vi "SiPM_Data_Analysis.vi"() -> ()   [LabVIEW 2019]
uses:
  <vilib>/Utility/error.llb/DialogType.ctl
  SiPM_Tests_Global_Var.vi
  Data_Analysis_subvis/ESA_Data_Analysis_Global_VIs.vi
  <vilib>/Analysis/NI_AALPro.lvlib
panel:
  out "property names":string[](array[string])
  out "property values":variant[](array[variant])
  out "data":waveform(dbl)[](array[waveform])
  out "Indicator":bool
  in  "Close Session":bool
  in  "Channel Selection":T1(ring)=enum."Channel 6"
  in  "Waveform Nb":u16
  in  "NbSamples":i64=1000000 caption="Nb of Samples to Analyze" format="%.0p"
  in  "Refresh":bool
  in  "Load file to display":bool
  in  "Detailed":bool
  in  "Listbox":i32[](listbox) caption="PIFN_ReadoutBoard.tdms"
  in  "CH6 Trigger Logic":T2(ring)=enum."Don't Care"
  in  "CH6 Trigger Thr":u16 caption="CH6 Trigger Thr (V)" step=1
  in  "CH5 Trigger Logic":T2(ring)=enum."Don't Care"
  in  "CH5 Trigger":u16 caption="CH5 Trigger Thr (V)" step=1
  in  "Tab Control":enum32{"Waveform", "Calibration"}(tab)
  out "Spectrum":u16[][](graph)
  in  "X-Scale":bool
  in  "Calibrate":bool
  out "Offset":dbl step=0.001 format="%#_6p"
  out "Gain":dbl step=0.001 format="%#_6p"
  in  "Y2 (keV)":dbl
  in  "Y1 (keV)":dbl
  in  "AutoScale 4":bool
  out "Waveform Graph":dbl[][](graph)
  in  "Lower Cut-Off":dbl=0.01
  in  "Y-Scale 2":bool caption="Y-Scale"
  in  "CH1 Trigger Logic":T2(ring)=enum."Don't Care"
  in  "CH1 Trigger Thr":u16 caption="CH1 Trigger Thr (V)" step=1
  in  "Y-Scale":bool
  out "Nb of Selected Events":dbl step=0.001 format="%#_6p"
  out "Total Nb of Recorded Events":dbl step=0.001 format="%#_6p"
  in  "CH4 Trigger Logic":T2(ring)=enum."Don't Care"
  in  "CH4 Trigger Thr":u16 caption="CH4 Trigger Thr (V)" step=1
  in  "CH3 Trigger Logic":T2(ring)=enum."Don't Care"
  in  "CH3 Trigger":u16 caption="CH3 Trigger Thr (V)" step=1
  in  "CH2 Trigger Logic":T2(ring)=enum."Don't Care"
  in  "CH2 Trigger Thr":u16 caption="CH2 Trigger Thr (V)" step=1
  in  "AutoScale 3":bool
  in  "Update Energy":bool
  out "Energy_Spectr":u16[][](graph)
  in  "Filter \nON?":bool
  in  "Threshold 2":dbl caption="Max_Value (V)" step=0.001 format="%#_6p"
  in  "Threshold":dbl caption="Energy Threshold (V)" step=0.001 format="%#_6p"
  out "Table":string[][](table)
  out "Nb of Channels in Group":i32
  out "group names":string[](array[string])
  out "tdms file out":refnum<k34>
  in  "File contents":string[](tree)
  # "NCSR  DEMOKRITOS\nInstitute of Nuclear and Particle Physics\nDetectors Instrumentation Laboratory"
  # "SiPM Data Analysis"
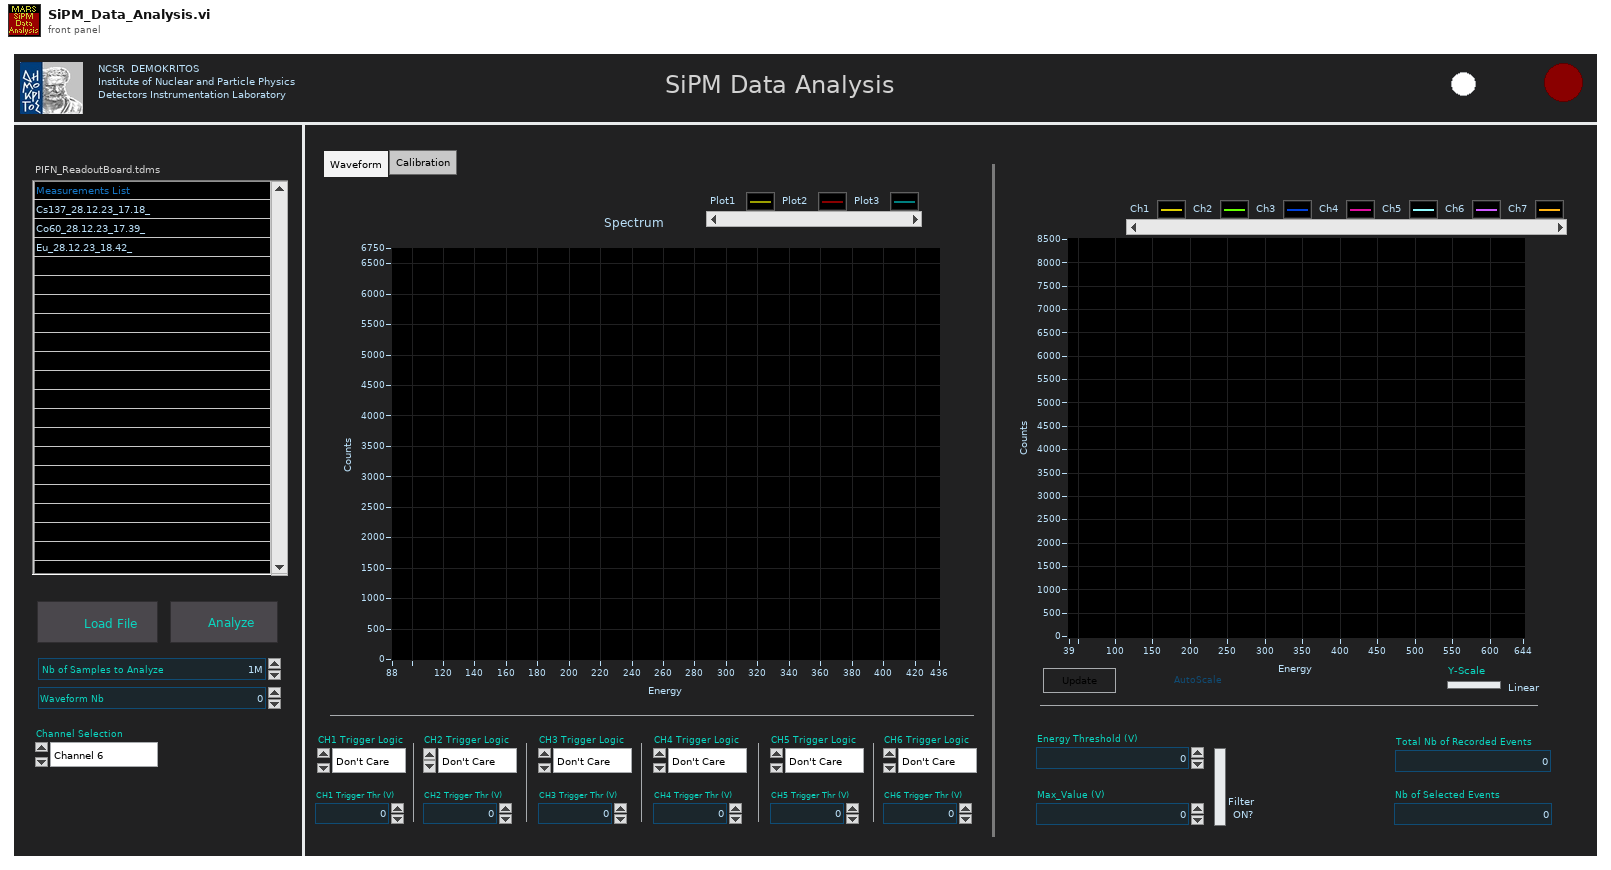
[diagram p1: front panel]
types:
  T1 = enum16{"Channel 1", "Channel 2", "Channel 3", "Channel 4", "Channle 5", "Channel 6", "Added Spectrum"}
  T2 = enum16{"Coincidence", "Anti-Coincidence", "Don't Care"}
  T3 = typedef "DialogType.ctl" = u16
  T4 = enum16{"open", "open or create", "create or replace", "create", "open (read-only)"}
  T5 = cluster{"X Values":dbl[], "Histogram: h(x)":i32[]}
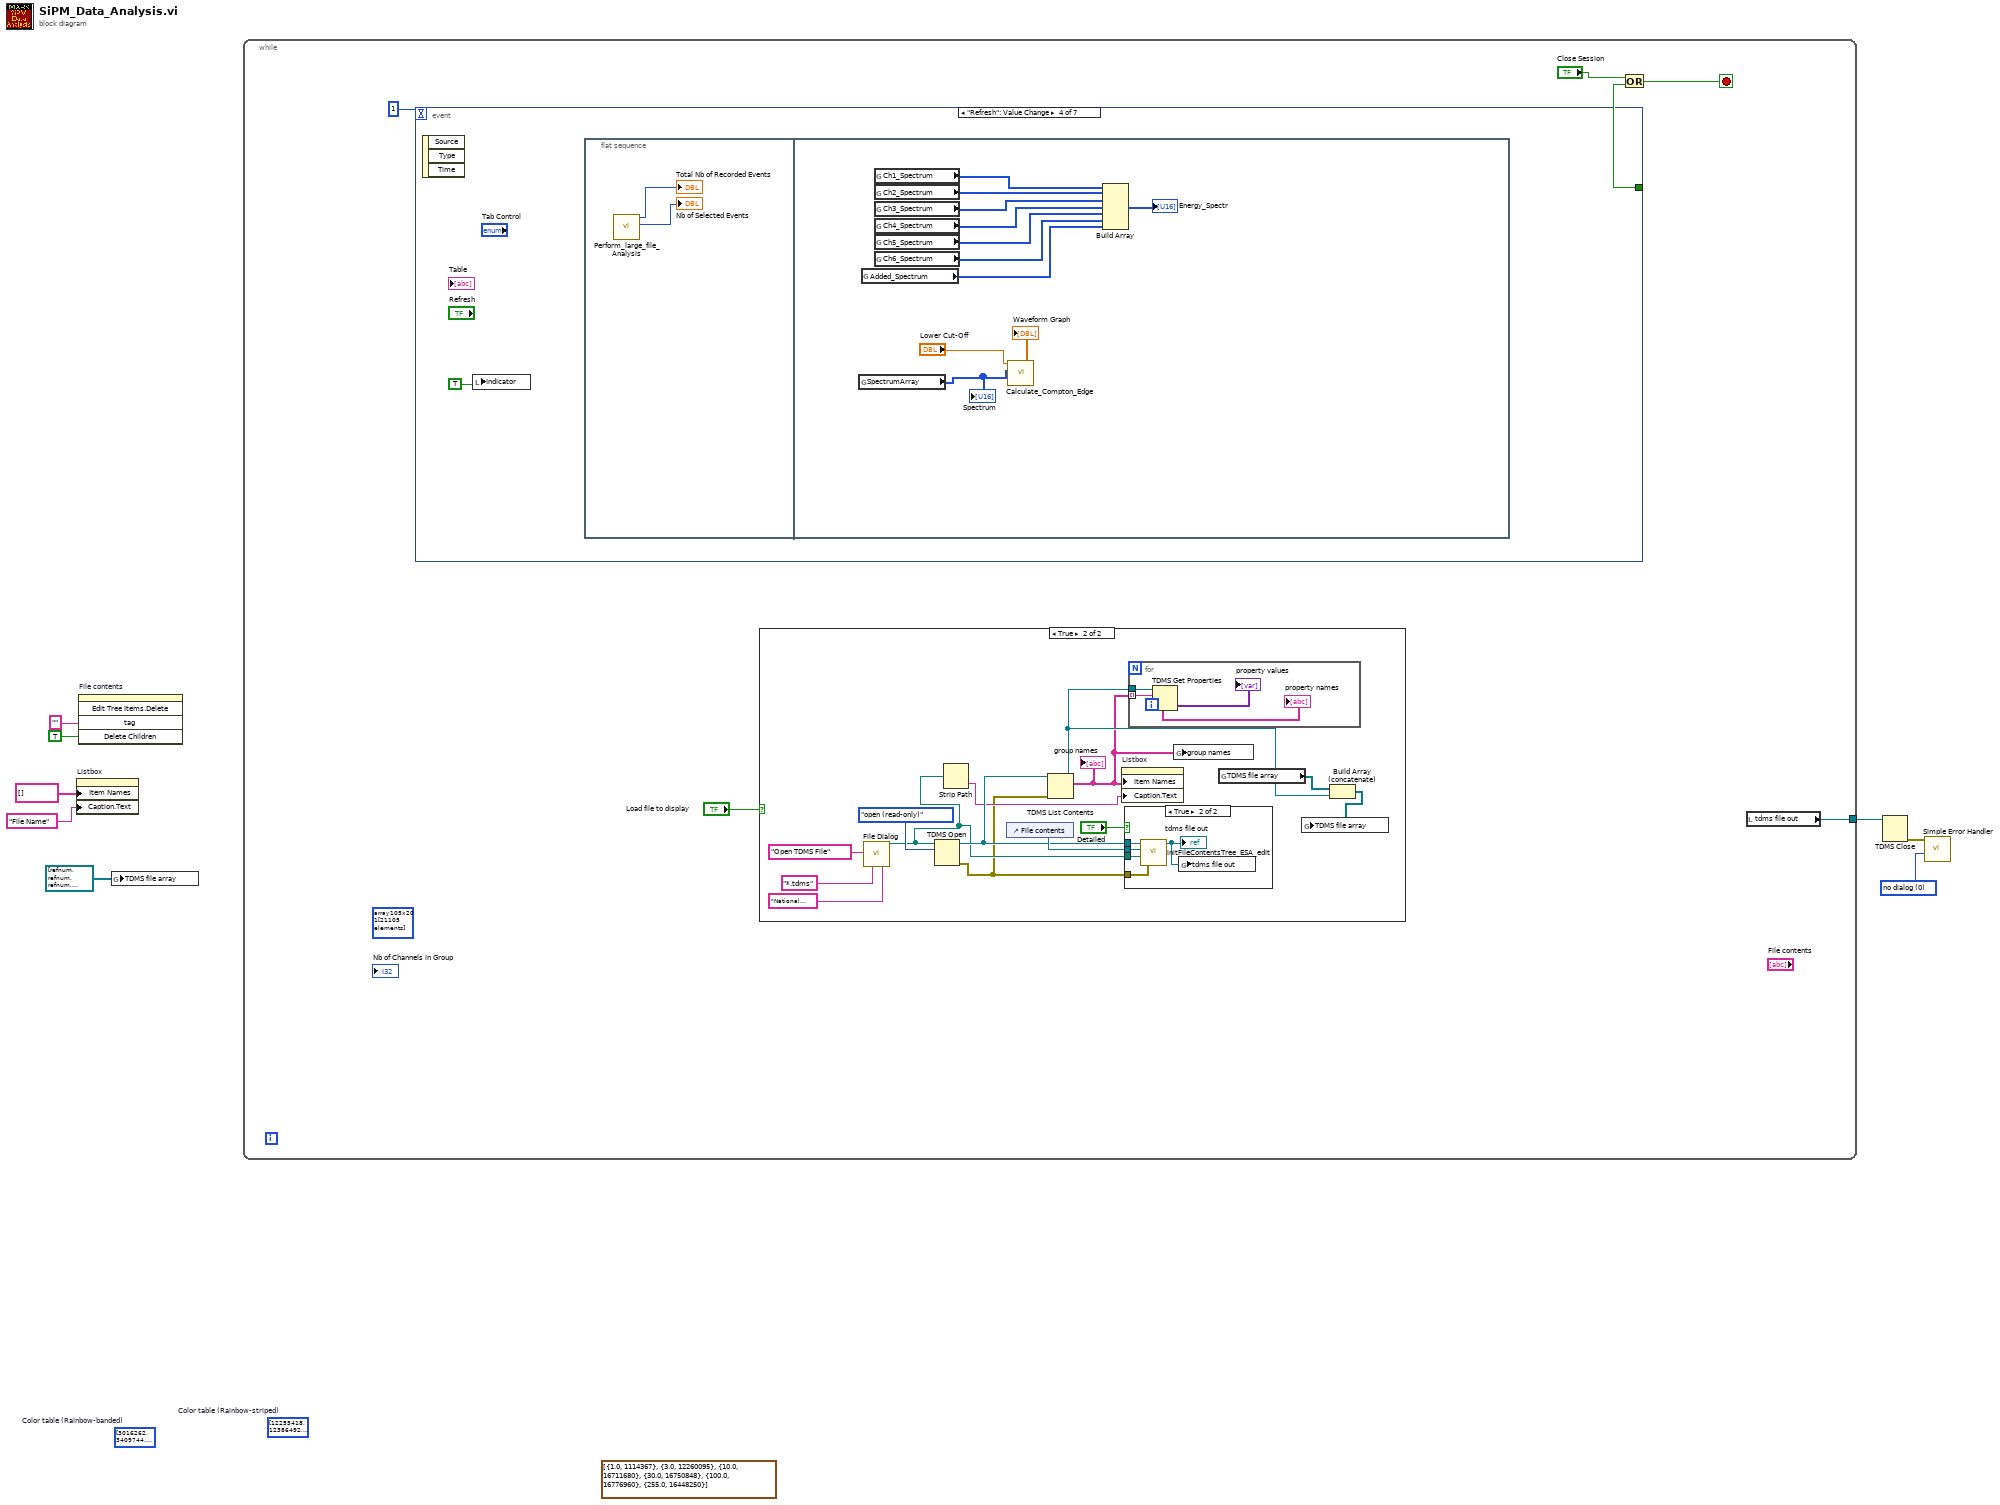
[diagram p0: block diagram]
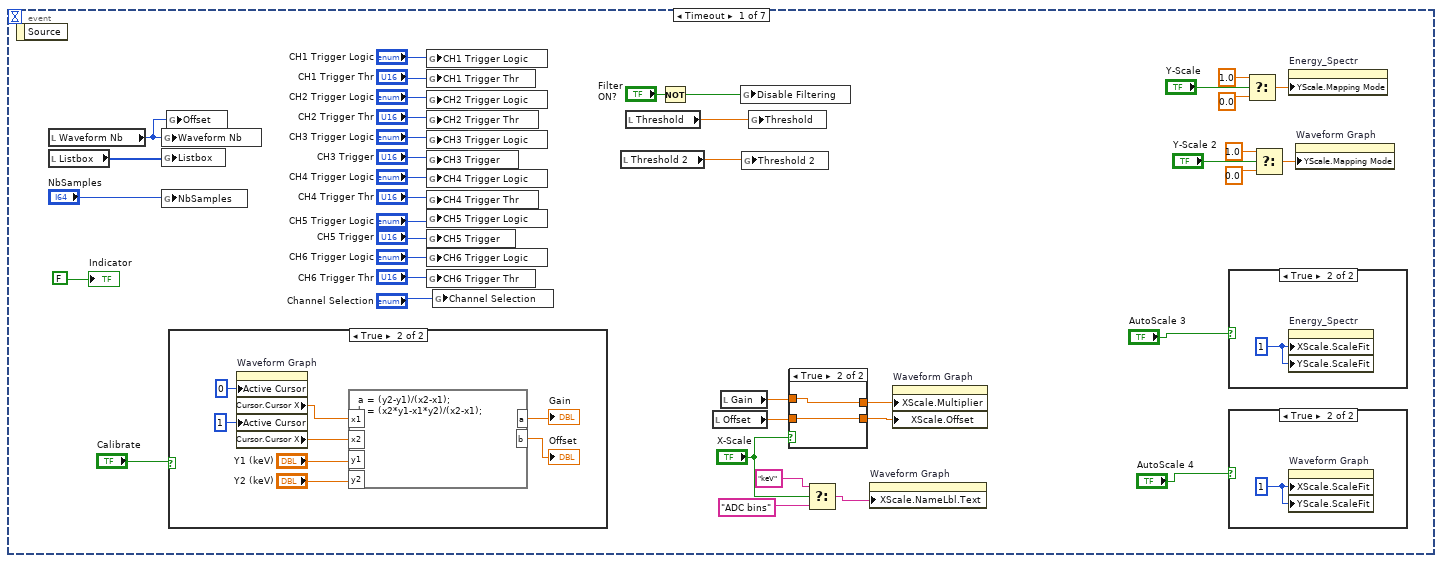
[diagram p2: hidden frame]
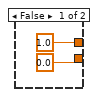
[diagram p3: hidden frame]
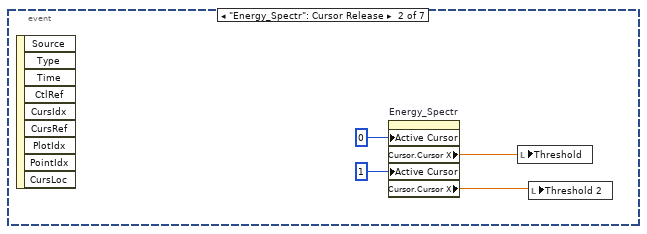
[diagram p7: hidden frame]
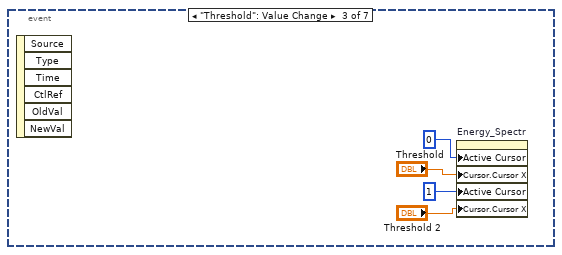
[diagram p8: hidden frame]
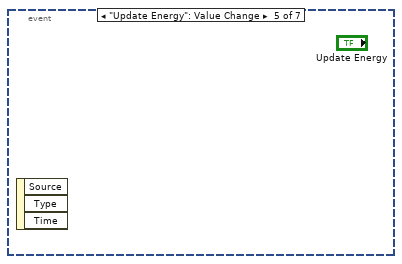
[diagram p9: hidden frame]
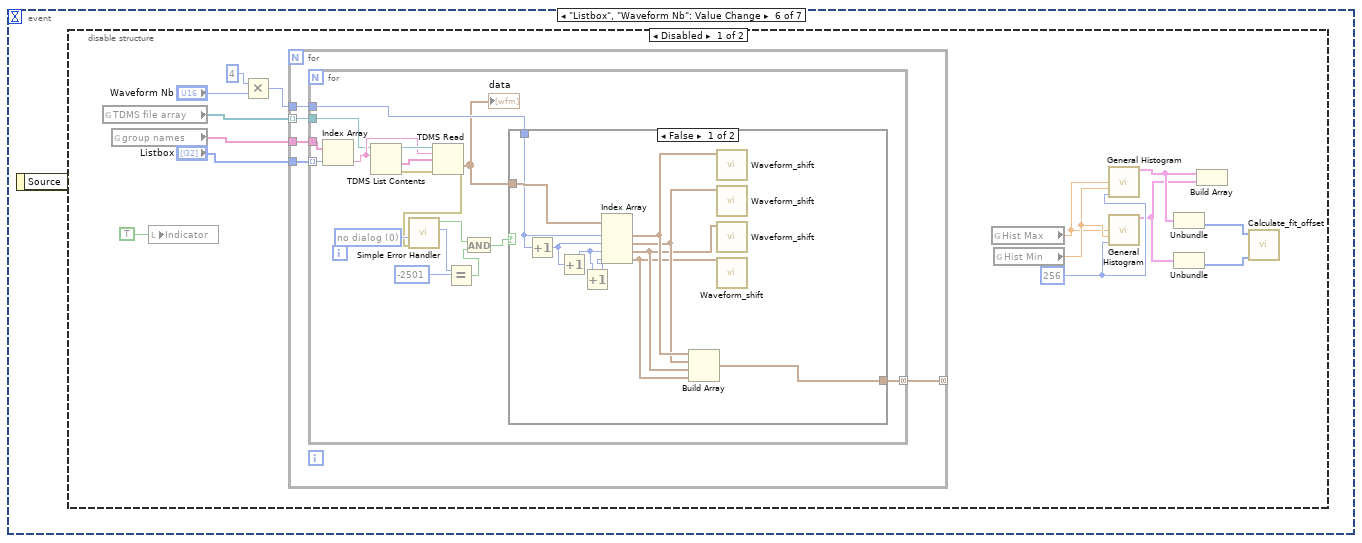
[diagram p10: hidden frame]
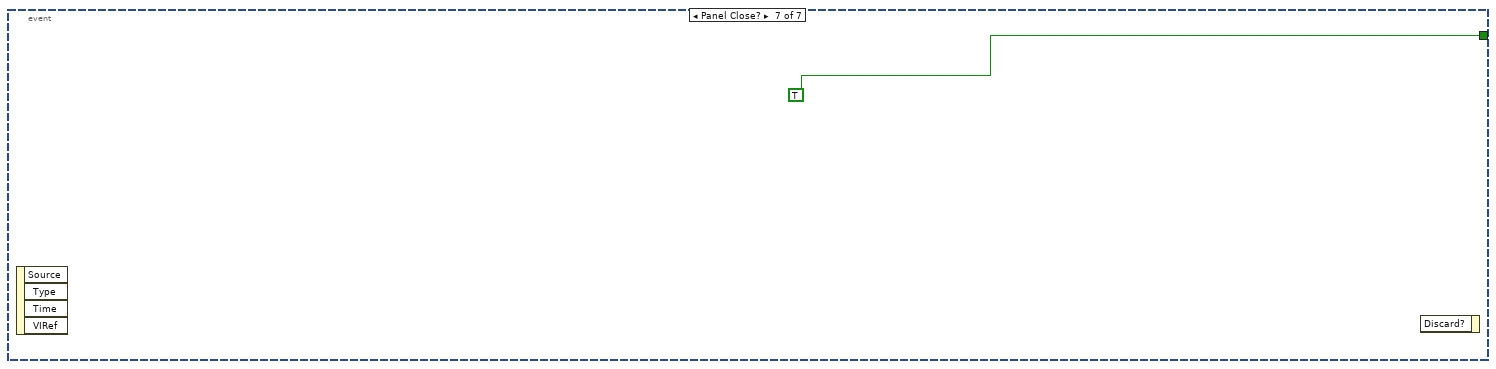
[diagram p13: hidden frame]
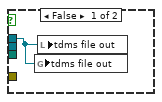
[diagram p15: hidden frame]
diagram:
  w1 = T3 0 items=["no dialog", "OK message", "continue or stop message", "OK message + warnings", "continue/stop + warnings"] ("type of dialog (OK msg:1)")
  (unwired) cluster{dbl, u32}[] [{1.0, 1114367}, {3.0, 12260095}, {10.0, 16711680}, {30.0, 16750848}, {100.0, 16776960}, {255.0, 16448250}] ("Z Scale.Marker Values[]")
  (unwired) u32[] [12255418, 12386492, 12517567, 12320960, 12189888, 12058817, 11927746, 11731139, 11600067, 9175197, 9044125, 11141318, 11010246, 10813639, 10682568, 10551497, 10354890, 10223818, 10092747, 7930019, 7798948, 9633997, 9502926, 9306319, 9175248, 9044176, 8847569, 8716498, 8585427, 6750377, 6619306, 8126677, 7995606, 7798999, 7667927, 7536856, 7340249, 7209178, 7078106, 5505199, 5374128, 6619357, 6488285, 6291678, 6160607, 6029536, 5832929, 5701857, 5570786, 4325557, 4194486, 5112036, 4980965, 4784358, 4653287, 4522215, 4325608, 4194537, 4063466, 3080380, 3014844, 3604716, 3408109, 3277038, 3277038, 3145966, 3014895, 2818288, 2687217, 2556145, 1900738, 1769666, 2097396, 1900789, 1769717, 1638646, 1507575, 1310968, 1179896, 1048825, 721096, 590024, 590075, 393468, 262397, 131326, 255, 1791, 3327, 4863, 5068, 6348, 9471, 11007, 12543, 14079, 15615, 17151, 18687, 20223, 17612, 18636, 25087, 26623, 28159, 29695, 31231, 32767, 34303, 35839, 29900, 31180, 40447, 41983, 43775, 45311, 46847, 48383, 49919, 51455, 42444, 43724, 56063, 57599, 59135, 60671, 62207, 63743, 65535, 65528, 52418, 52413, 65510, 65504, 65498, 65492, 65486, 65480, 65474, 65468, 52369, 52364, 65449, 65443, 65437, 65431, 65425, 65419, 65413, 65407, 52321, 52316, 65389, 65383, 65377, 65371, 65364, 65358, 65352, 65346, 52272, 52267, 65328, 65322, 65316, 65310, 65304, 65298, 65292, 65286, 52224, 314368, 851712, 1244928, 1638144, 2031360, 2424576, 2817792, 3211008, 3604224, 3197952, 3525632, 4783872, 5177088, 5635840, 6029056, 6422272, 6815488, 7208704, 7601920, 6409216, 6736896, 6736896, 8781568, 9174784, 9568000, 9961216, 10354432, 10747648, 11206400, 11599616, 9554944, 9882624, 12779264, 13172480, 13565696, 13958912, 14352128, 14745344, 15138560, 15531776, 12766208, 13093888, 16776960, 16775170, 16773637, 16771847, 16770314, 16768780, 16766991, 16765457, 13411088, 13409810, 16760601, 16758812, 16757278, 16755745, 16753955, 16752422, 16750888, 16749099, 13398052, 13396774, 16744243, 16742704, 16741166, 16739884, 16738345, 16736807, 16735269, 16733730, 13385753, 13384728, 16729371, 16727833, 16726295, 16725012, 16723474, 16721936, 16720397, 16718859, 13373959, 13372677, 16714500, 16712962, 16711680]  # Color table (Rainbow-striped)
  (unwired) u32[] [3016262, 3409744, 4000097, 4721526, 5508493, 6229924, 6820281, 7214025, 7345364, 7279831, 6886611, 6362057, 5640632, 4788132, 4001165, 3214197, 2492769, 2033488, 1640006, 1508930, 1508934, 1640272, 1902945, 2165622, 2428301, 2690980, 2822585, 2888649, 2757844, 2626775, 2299091, 1971145, 1642936, 1249188, 920973, 724086, 592737, 461392, 395846, 396098, 396358, 462928, 595297, 727925, 861069, 994212, 1127608, 1260745, 1328083, 1329111, 1329876, 1264073, 1132217, 999844, 866957, 734070, 600929, 468304, 401734, 401730, 402502, 469584, 603489, 737909, 737909, 872845, 1008036, 1143224, 1277641, 1345747, 1347287, 1347796, 1281225, 1147833, 1013668, 878989, 743798, 609121, 475216, 407878, 407362, 408390, 476496, 611681, 747893, 884877, 1022116, 1158840, 1294793, 1363667, 1365719, 1365202, 1296836, 1161649, 1025178, 888194, 751211, 614742, 479302, 411196, 410168, 411193, 479297, 614732, 750939, 888171, 1025145, 1161350, 1296782, 1364883, 1365906, 1365132, 1296769, 1161588, 1025124, 888147, 751172, 614710, 479276, 411173, 410146, 411170, 479270, 614700, 750900, 888124, 1025091, 1161289, 1296716, 1364813, 1365834, 1365062, 1296703, 1161527, 1025070, 888101, 751133, 614678, 479249, 411149, 410124, 411147, 479244, 614668, 750861, 888078, 1156111, 1488913, 1820947, 2151188, 2414356, 2610196, 2738451, 2668817, 2597903, 2329869, 2061835, 1794313, 1593351, 1459718, 1458694, 1590790, 1921031, 2449673, 3110155, 3902733, 4695055, 5486609, 6211859, 6738708, 7132948, 7197716, 7063827, 6666513, 6136847, 5410061, 4617739, 3957001, 3362823, 2967046, 2900486, 3098118, 3690503, 4546825, 5666059, 6917389, 8233999, 9484305, 10537235, 11326228, 11786004, 11785236, 11785236, 11454739, 10729745, 9675791, 8424717, 7173643, 6054153, 5066759, 4474374, 4342278, 4605190, 5262855, 6380553, 7695883, 9273613, 10785807, 12100625, 13217555, 13874452, 14136340, 13938196, 13214227, 12161553, 10780431, 9267725, 7755531, 6374921, 5257479, 4599814, 4336646, 4599302, 5255943, 6372361, 7685899, 9261837, 10771983, 12085009, 13200659, 13856532, 14118164, 13920276, 13197075, 12145937, 10766351, 9255949, 7745547, 6366729, 5250567, 4593926, 4331014, 4593158, 5249287, 6364169, 7675915, 9249805, 10758159, 12069393, 13183507, 13838612, 14099988, 13902356, 13180179, 12130065, 10752527]  # Color table (Rainbow-banded)
  n1 = property on="Listbox" class="LstBox (strict)"("Item Names"=string[] [], "Caption.Text"="File Name") -> ()  [unwired: 2 in, 2 out]
  n2 = invoke on="File contents" class="Tree (strict)" method="Edit Tree Items.Delete"("tag"="" ("Tag"), "Delete Children"=TRUE ("Delete Children?")) -> ()  [unwired: 3 in, 5 out]
  n3 = global write "SiPM_Tests_Global_Var.vi" "TDMS file array"(refnum<k34>[] [refnum, refnum, refnum, refnum] ("TDMS file array")) -> ()
  n4 = while {
    tunnel: [w13] -> w8
    stop <- w12 stop-if-true
    (unwired) i32[][] array105x201[21105 elements] ("spectrum")
    n5 = event shown="[3] \"Refresh\": Value Change" {
      selector: _ -> [_ _ _ _ _ _ _]
      dyn-events: _ -> [_ _ _ _ _ _ _]
      timeout: 1 -> [_ _ _ _ _ _ _]
      tunnel: [_ _ _ _ _ _ TRUE ("Stop Button")] -> w11
      event Timeout {
        n6 = event-data() -> ()  [unwired: 1 in, 1 out]
        n7 = local read "Waveform Nb"() -> (w15:u16)
        n8 = local read "Listbox"() -> (w53:i32[])
        n9 = global write "SiPM_Tests_Global_Var.vi" "Waveform Nb"(w15) -> ()
        n10 = global write "ESA_Data_Analysis_Global_VIs.vi" "Listbox"(w53) -> ()
        n11 = global write "SiPM_Tests_Global_Var.vi" "NbSamples"("NbSamples") -> ()
        n12 = global write "SiPM_Tests_Global_Var.vi" "Offset"(w15) -> ()
        n13 = case shown="True" "Calibrate" {
          frame False {
          }
          frame True {
            n14 = property on="Waveform Graph" class="WFGraph (strict)"("Active Cursor"=u32 0, "Active Cursor"=u32 1) -> ("Cursor.Cursor X"=w64:dbl, "Cursor.Cursor X"=w63:dbl)  [unwired: 2 in, 2 out]
            n15 = formula code="a = (y2-y1)/(x2-x1);\nb = (x2*y1-x1*y2)/(x2-x1);"("x1"=w64, "x2"=w63, "y1"="Y1 (keV)", "y2"="Y2 (keV)") -> ("a"=→"Gain":dbl, "b"=→"Offset":dbl)
          }
        }
        n16 = global write "SiPM_Tests_Global_Var.vi" "CH1 Trigger Logic"("CH1 Trigger Logic") -> ()
        n17 = global write "SiPM_Tests_Global_Var.vi" "CH1 Trigger Thr"("CH1 Trigger Thr") -> ()
        n18 = global write "SiPM_Tests_Global_Var.vi" "CH2 Trigger Logic"("CH2 Trigger Logic") -> ()
        n19 = global write "SiPM_Tests_Global_Var.vi" "CH2 Trigger Thr"("CH2 Trigger Thr") -> ()
        n20 = global write "SiPM_Tests_Global_Var.vi" "CH3 Trigger Logic"("CH3 Trigger Logic") -> ()
        n21 = global write "SiPM_Tests_Global_Var.vi" "CH3 Trigger"("CH3 Trigger") -> ()
        n22 = global write "SiPM_Tests_Global_Var.vi" "CH4 Trigger Logic"("CH4 Trigger Logic") -> ()
        n23 = global write "SiPM_Tests_Global_Var.vi" "CH4 Trigger Thr"("CH4 Trigger Thr") -> ()
        n24 = global write "SiPM_Tests_Global_Var.vi" "CH5 Trigger Logic"("CH5 Trigger Logic") -> ()
        n25 = global write "SiPM_Tests_Global_Var.vi" "CH5 Trigger"("CH5 Trigger") -> ()
        n26 = global write "SiPM_Tests_Global_Var.vi" "CH6 Trigger Logic"("CH6 Trigger Logic") -> ()
        n27 = global write "SiPM_Tests_Global_Var.vi" "CH6 Trigger Thr"("CH6 Trigger Thr") -> ()
        n28 = global write "SiPM_Tests_Global_Var.vi" "Channel Selection"("Channel Selection") -> ()
        n29 = local read "Threshold 2"() -> (w50:dbl)
        n30 = local read "Threshold"() -> (w51:dbl)
        n31 = Not(x="Filter \nON?") -> (.not. x?=w48:bool)
        n32 = local read "Offset"() -> (w25:dbl)
        n33 = local read "Gain"() -> (w26:dbl)
        n34 = global write "SiPM_Tests_Global_Var.vi" "Disable Filtering"(w48) -> ()
        n35 = global write "SiPM_Tests_Global_Var.vi" "Threshold 2"(w50) -> ()
        n36 = global write "SiPM_Tests_Global_Var.vi" "Threshold"(w51) -> ()
        n37 = case shown="True" "X-Scale" {
          tunnel: [1.0 ("gain") w58] -> w28
          tunnel: w26 -> [_ w58]
          tunnel: [0.0 ("offset") w57] -> w27
          tunnel: w25 -> [_ w57]
          frame False {
          }
          frame True {
          }
        }
        n38 = Select(t="keV" ("X Scale.Unit Label.Text"), s="X-Scale", f="ADC bins" ("X Scale.Unit Label.Text")) -> (s? t:f=w21:string)
        n39 = property on="Waveform Graph" class="WFGraph (strict)"("XScale.NameLbl.Text"=w21) -> ()  [unwired: 2 in, 2 out]
        n40 = property on="Waveform Graph" class="WFGraph (strict)"("XScale.Multiplier"=w28, "XScale.Offset"=w27) -> ()  [unwired: 2 in, 2 out]
        n41 = case shown="True" "AutoScale 3" {
          frame False {
          }
          frame True {
            w67 = u8 1 ("X Scale.Scale Fit")
            n42 = property on="Energy_Spectr" class="WFGraph (strict)"("XScale.ScaleFit"=w67, "YScale.ScaleFit"=w67) -> ()  [unwired: 2 in, 2 out]
          }
        }
        n43 = case shown="True" "AutoScale 4" {
          frame False {
          }
          frame True {
            w68 = u8 1 ("X Scale.Scale Fit")
            n44 = property on="Waveform Graph" class="WFGraph (strict)"("XScale.ScaleFit"=w68, "YScale.ScaleFit"=w68) -> ()  [unwired: 2 in, 2 out]
          }
        }
        n45 = Select(t=1.0, s="Y-Scale", f=0.0 ("t")) -> (s? t:f=w41:dbl)
        n46 = Select(t=1.0, s="Y-Scale 2", f=0.0 ("t")) -> (s? t:f=w33:dbl)
        n47 = property on="Energy_Spectr" class="WFGraph (strict)"("YScale.Mapping Mode"=w41) -> ()  [unwired: 2 in, 2 out]
        n48 = property on="Waveform Graph" class="WFGraph (strict)"("YScale.Mapping Mode"=w33) -> ()  [unwired: 2 in, 2 out]
        "Indicator" <- FALSE ("Indicator")
      }
      event "Energy_Spectr": Cursor Release {
        n49 = event-data() -> ()  [unwired: 1 in, 9 out]
        n50 = property on="Energy_Spectr" class="WFGraph (strict)"("Active Cursor"=u32 0, "Active Cursor"=u32 1) -> ("Cursor.Cursor X"=w72:dbl, "Cursor.Cursor X"=w69:dbl)  [unwired: 2 in, 2 out]
        n51 = local write "Threshold"(w72) -> ()
        n52 = local write "Threshold 2"(w69) -> ()
      }
      event "Threshold": Value Change {
        n53 = event-data() -> ()  [unwired: 1 in, 6 out]
        n54 = property on="Energy_Spectr" class="WFGraph (strict)"("Active Cursor"=u32 0, "Cursor.Cursor X"="Threshold", "Active Cursor"=u32 1, "Cursor.Cursor X"="Threshold 2") -> ()  [unwired: 2 in, 2 out]
      }
      event "Refresh": Value Change {
        n55 = event-data() -> ()  [unwired: 1 in, 3 out]
        n56 = local write "Indicator"(TRUE ("Indicator")) -> ()
        n57 = flat-sequence {
          frame #0 {
            n58 = call "Perform_large_file_Analysis.vi"() -> ("Filtered Nb of Events"=→"Nb of Selected Events":i32, "Total Nb of Events"=→"Total Nb of Recorded Events":i32)  [unwired: 7 in]
          }
          frame #1 {
            n59 = global read "SiPM_Tests_Global_Var.vi" "SpectrumArray"() -> (w80:u16[][])
            "Spectrum" <- w80
            n60 = global read "SiPM_Tests_Global_Var.vi" "Added_Spectrum"() -> (w82:u16[])
            n61 = global read "SiPM_Tests_Global_Var.vi" "Ch1_Spectrum"() -> (w88:u16[])
            n62 = global read "SiPM_Tests_Global_Var.vi" "Ch2_Spectrum"() -> (w87:u16[])
            n63 = global read "SiPM_Tests_Global_Var.vi" "Ch3_Spectrum"() -> (w86:u16[])
            n64 = global read "SiPM_Tests_Global_Var.vi" "Ch4_Spectrum"() -> (w85:u16[])
            n65 = global read "SiPM_Tests_Global_Var.vi" "Ch5_Spectrum"() -> (w84:u16[])
            n66 = global read "SiPM_Tests_Global_Var.vi" "Ch6_Spectrum"() -> (w83:u16[])
            n67 = call "Calculate_Compton_Edge.vi"("Spectrum_Array"=w80, "Lower Cut-Off"="Lower Cut-Off") -> ("Waveform Graph"=→"Waveform Graph":dbl[][])  [unwired: 9 in]
            n68 = Build Array(w88, w87, w86, w85, w84, w83, w82) -> (→"Energy_Spectr":u16[][])
          }
        }
      }
      event "Update Energy": Value Change {
        n69 = event-data() -> ()  [unwired: 1 in, 3 out]
      }
      event "Listbox", "Waveform Nb": Value Change {
        n70 = event-data() -> ()  [unwired: 1 in, 1 out]
        n71 = disable-structure shown="Disabled" {
          frame Disabled {
            w95 = 256 ("# bins")
            n72 = global read "SiPM_Tests_Global_Var.vi" "TDMS file array"() -> (w103:refnum<k34>[])
            n73 = global read "ESA_Data_Analysis_Global_VIs.vi" "group names"() -> (w104:string[])
            n74 = local write "Indicator"(TRUE ("Indicator")) -> ()
            n75 = Multiply(x=4, y="Waveform Nb") -> (x*y=w99:i32)
            n76 = for {
              tunnel: "Listbox" -> [w109]
              tunnel: w104 -> [w108]
              tunnel: w103 -> [w107] mode=indexing
              tunnel: [w106] -> _ mode=concatenating
              tunnel: w99 -> [w105]
              n77 = for {
                tunnel: w109 -> [w122] mode=indexing
                tunnel: w108 -> [w121]
                tunnel: w107 -> [w120]
                tunnel: [w119] -> w106 mode=concatenating
                tunnel: w105 -> [w111]
                w118 = T3 0 items=["no dialog", "OK message", "continue or stop message", "OK message + warnings", "continue/stop + warnings"] ("type of dialog (OK msg:1)")
                n78 = Index Array(array=w121, index=w122) -> (element=w125:string)
                n79 = TDMS List Contents(6:w125, 7:w120) -> (0:w123:errorcluster, 1:w124:string[], 3:w126:refnum<k34>)  [unwired: 1 in, 1 out]
                n80 = TDMS Read(0:w126, 5:w125, 7:w124, 11:w123) -> (10:w110:waveform(dbl)[], 15:w114:errorcluster)  [unwired: 4 in, 4 out]
                "data" <- w110
                n81 = call <vilib>:"Simple Error Handler.vi"("type of dialog (OK msg:1)"=w118, "error in (no error)"=w114) -> ("error?"=w113:bool, "code out"=w117:i32)  [unwired: 3 in, 3 out]
                n82 = Equal?(x=w117, y=-2501) -> (x = y?=w115:bool)
                n83 = And(x=w113, y=w115) -> (x .and. y?=w112:bool)
                n84 = case shown="False" w112 {
                  tunnel: w110 -> [w136 _]
                  tunnel: [w132 _] -> w119
                  tunnel: w111 -> [w135 _]
                  frame False {
                    n85 = Increment(x=w135) -> (x+1=w131:i32)
                    n86 = Increment(x=w131) -> (x+1=w129:i32)
                    n87 = Increment(x=w129) -> (x+1=w130:i32)
                    n88 = Index Array(array=w136, index #1=w135, index #2=w131, index #3=w129, index #4=w130) -> (element #1=w134:waveform(dbl), element #2=w133:waveform(dbl), element #3=w128:waveform(dbl), element #4=w127:waveform(dbl))
                    n89 = Build Array(w134, w133, w128, w127) -> (w132:waveform(dbl)[])
                    n90 = call "Waveform_shift.vi"("Waveform_in"=w134) -> ()  [unwired: 9 in, 1 out]
                    n91 = call "Waveform_shift.vi"("Waveform_in"=w133) -> ()  [unwired: 9 in, 1 out]
                    n92 = call "Waveform_shift.vi"("Waveform_in"=w128) -> ()  [unwired: 9 in, 1 out]
                    n93 = call "Waveform_shift.vi"("Waveform_in"=w127) -> ()  [unwired: 9 in, 1 out]
                  }
                  frame True {
                  }
                }
              }
            }
            n94 = global read "SiPM_Tests_Global_Var.vi" "Hist Max"() -> (w96:dbl)
            n95 = global read "SiPM_Tests_Global_Var.vi" "Hist Min"() -> (w97:dbl)
            n96 = call <vilib>:"General Histogram.vi"("max"=w96, "min"=w97, "# bins"=w95) -> ("Histogram Graph"=w94:T5)  [unwired: 8 in, 4 out]
            n97 = call <vilib>:"General Histogram.vi"("max"=w96, "min"=w97, "# bins"=w95) -> ("Histogram Graph"=w93:T5)  [unwired: 8 in, 4 out]
            n98 = Unbundle(w94) -> ("Histogram: h(x)"=w92:i32[])  [unwired: 1 out]
            n99 = Unbundle(w93) -> ("Histogram: h(x)"=w91:i32[])  [unwired: 1 out]
            n100 = Build Array(w94, w93) -> ()  [unwired: 1 out]
            n101 = call "Calculate_fit_offset.vi"("baseline1"=w92, "baseline2"=w91) -> ()  [unwired: 4 in, 4 out]
          }
          frame Enabled {
          }
        }
      }
      event Panel Close? {
        n102 = event-data() -> ()  [unwired: 1 in, 4 out]
        n103 = event-data() -> ()  [unwired: 2 in, 1 out]
      }
    }
    n104 = case shown="True" "Load file to display" {
      frame False {
      }
      frame True {
        n105 = call "File Dialog"("prompt"="Open TDMS File" ("prompt tdms"), "pattern (all files)"="*.tdms", "pattern label"="National Instruments TDM Streaming" ("pattern label tdms")) -> ("selected path"=w145:path)  [unwired: 4 in, 8 out]
        n106 = TDMS Open(10:T4."open (read-only)" ("operation (0:open)"), 11:w145) -> (0:w142:errorcluster, 3:w146:refnum<k34>)  [unwired: 5 in]
        n107 = Strip Path(path=w145) -> (name=w144:string)  [unwired: 1 out]
        n108 = control-ref of="File contents"() -> (w151:refnum<vi>)
        n109 = TDMS List Contents(4:w142, 7:w146) -> (2:w138:string[], 3:w139:refnum<k34>)  [unwired: 1 in, 2 out]
        "group names" <- w138
        n110 = property on="Listbox" class="LstBox (strict)"("Item Names"=w138, "Caption.Text"=w144) -> ()  [unwired: 2 in, 2 out]
        n111 = case shown="True" "Detailed" {
          tunnel: w151 -> [_ w161]
          tunnel: w142 -> [_ w160]
          tunnel: w145 -> [_ w159]
          tunnel: w146 -> [w156 w158]
          frame False {
            n112 = global write "ESA_Data_Analysis_Global_VIs.vi" "tdms file out"(w156) -> ()
            n113 = local write "tdms file out"(w156) -> ()
          }
          frame True {
            n114 = call "initFileContentsTree_ESA_edit.vi"("error in (no error)"=w160, "file path"=w159, "Tree Refnum"=w161, "tdms file"=w158) -> ("tdms file out"=w157:refnum<k34>)  [unwired: 2 in, 1 out]
            "tdms file out" <- w157
            n115 = global write "ESA_Data_Analysis_Global_VIs.vi" "tdms file out"(w157) -> ()
          }
        }
        n116 = for {
          tunnel: w139 -> [w155]
          tunnel: w138 -> [w152] mode=indexing
          n117 = TDMS Get Properties(10:w152, 11:w155) -> (4:→"property values":variant[], 6:→"property names":string[])  [unwired: 4 in, 4 out]
        }
        n118 = global write "ESA_Data_Analysis_Global_VIs.vi" "group names"(w138) -> ()
        n119 = global read "SiPM_Tests_Global_Var.vi" "TDMS file array"() -> (w141:refnum<k34>[])
        n120 = Build Array (concatenate)(w141, w139) -> (w140:refnum<k34>[])
        n121 = global write "SiPM_Tests_Global_Var.vi" "TDMS file array"(w140) -> ()
      }
    }
    n122 = Or(x="Close Session", y=w11) -> (x .or. y?=w12:bool)
    n123 = local read "tdms file out"() -> (w13:refnum<k34>)
  }
  n124 = TDMS Close(11:w8) -> (0:w2:errorcluster)  [unwired: 1 in, 1 out]
  n125 = call <vilib>:"Simple Error Handler.vi"("type of dialog (OK msg:1)"=w1, "error in (no error)"=w2) -> ()  [unwired: 3 in, 5 out]
